vi "Check Valid Message.vi"(8 "error in (no error)":errorcluster, 10 "Message":string, 11 "Temperature Controller in":refnum<class "Temperature Controller.lvclass">) -> (0 "error out":errorcluster, 2 "Valid?":bool, 3 "Temperature Controller out":refnum<class "Temperature Controller.lvclass">)   [LabVIEW 2020, in "Temperature Controller.lvclass"]
uses:
  Temperature Controller.lvclass
  Temperature Controller.lvclass/Temperature Controller.ctl
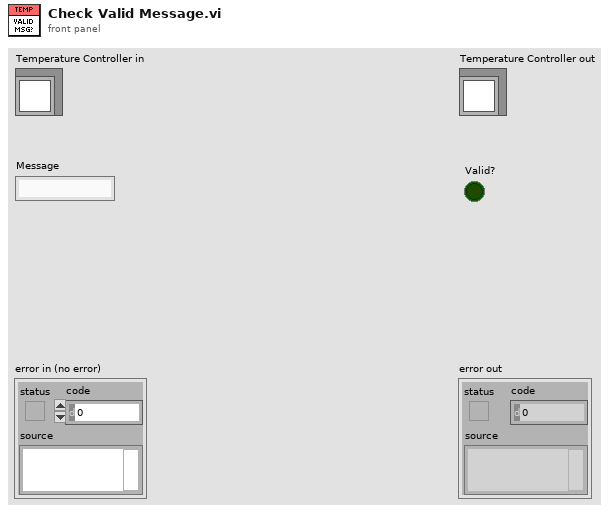
[diagram p1: front panel]
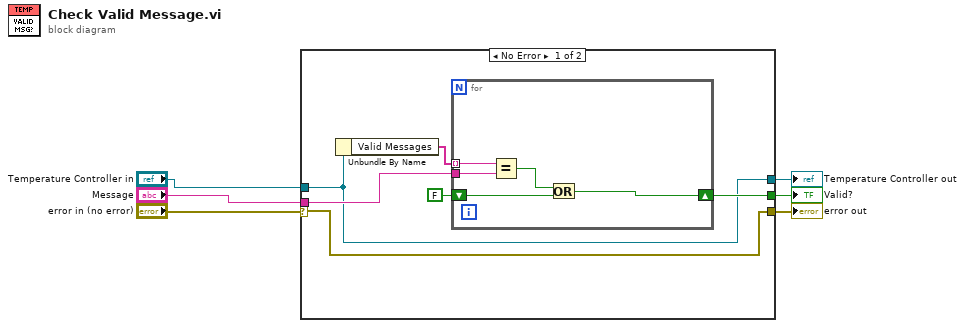
[diagram p0: block diagram]
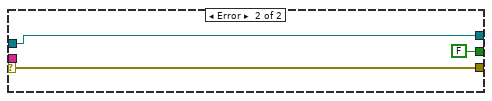
[diagram p2: hidden frame]
diagram:
  n1 = case shown="No Error" "error in (no error)" {
    selector: "error in (no error)" -> [w9 w19]
    tunnel: [w12 FALSE ("Valid?")] -> w5
    tunnel: "Temperature Controller in" -> [w8 w20]
    tunnel: "Message" -> [w11 _]
    tunnel: [w9 w19] -> w2
    tunnel: [w8 w20] -> w1
    frame No Error {
      n2 = Unbundle By Name(w8) -> ("Valid Messages"=w10:string[])
      n3 = for {
        tunnel: w10 -> [w16] mode=indexing
        tunnel: w11 -> [w17]
        shift-right: [w13] -> w12
        shift-left: FALSE -> [w14]
        n4 = Equal?(x=w16, y=w17) -> (x = y?=w15:bool)
        n5 = Or(x=w15, y=w14) -> (x .or. y?=w13:bool)
      }
    }
    frame Error {
    }
  }
  "error out" <- w2
  "Temperature Controller out" <- w1
  "Valid?" <- w5
